vi "WLAN - niVST - OPPO - RFSG - Create and Down Load Wfm.vi"(0 "instrument handle":refnum<k15>="pxi1slot2", 1 "Waveform Generation Settings":T2 {"DSSS Data Rate (Mbps)" items=["1", "2", "5.5 CCK", "5.5 PBCC", "11 CCK", "11 PBCC", "22", "33"]; "OFDM Data Rate (Mbps)" items=["6", "9", "12", "18", "24", "36", "48", "54"]; "80211n PLCP Frame Format" items=["Mixed Format", "Greenfield Format"]; "Standard" items=["80211A/G/J/P OFDM", "80211B/G DSSS", "80211G DSSSOFDM", "80211N MIMOOFDM", "80211AC MIMOOFDM"]}, 5 "WaveformNamePostfix":string, 11 "error in":errorcluster, 12 "Address String":string="00:90:4C:C5:12:38") -> (4 "instrument handle":refnum<k15>, 6 "Rx_Test Parameters":T1 {"OFDM Data Rate (Mbps)" items=["6", "9", "12", "18", "24", "36", "48", "54"]; "DSSS Data Rate (Mbps)" items=["1", "2", "5.5 CCK", "5.5 PBCC", "11 CCK", "11 PBCC", "22", "33"]; "80211n PLCP Frame Format" items=["Mixed Format", "Greenfield Format"]}, 15 "error out":errorcluster)   [LabVIEW 2012]
uses:
  TV/RW/Includes/WLAN - TV - RW - INC - Rx_PER_Wfm_Settings.ctl
  TV/RW/Includes/WLAN - TV - RW - INC - RxTestParameters.ctl
  <instrlib>/niRFSG/niRFSG.llb/niRFSG Write Arb Waveform (Complex Input).vi
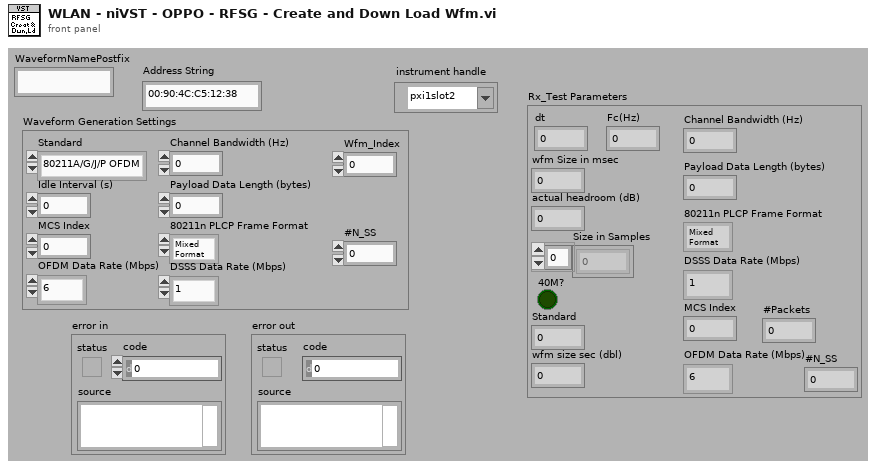
[diagram p1: front panel]
types:
  T1 = typedef "WLAN - TV - RW - INC - RxTestParameters.ctl" = cluster{"wfm Size in msec":i32, "actual headroom (dB)":dbl, "Size in Samples":i32[], "40M?":bool, "Standard ":i32, "wfm size sec (dbl)":dbl, "dt":dbl, "Channel Bandwidth (Hz)":dbl, "Payload Data Length (bytes)":i32, "80211n PLCP Frame Format":i32, "DSSS Data Rate (Mbps)":i32, "OFDM Data Rate (Mbps)":i32, "MCS Index":i32, "Fc(Hz)":dbl, "#Packets":i32, "#N_SS":i32}
  T2 = typedef "WLAN - TV - RW - INC - Rx_PER_Wfm_Settings.ctl" = cluster{"Standard":i32, "Channel Bandwidth (Hz)":dbl, "Idle Interval (s)":dbl, "MCS Index":i32, "80211n PLCP Frame Format":i32, "Payload Data Length (bytes)":i32, "OFDM Data Rate (Mbps)":i32, "DSSS Data Rate (Mbps)":i32, "Wfm_Index":i32, "#N_SS":i32}
  T3 = cluster{"Waveforms":cluster{"t0":dbl, "dt":dbl, "Y":cdb[]}[], "wfm Size in msec":i32, "actual headroom (dB)":dbl, "Size in Samples":i32[], "40M?":bool, "Standard ":i32, "wfm size sec (dbl)":dbl}
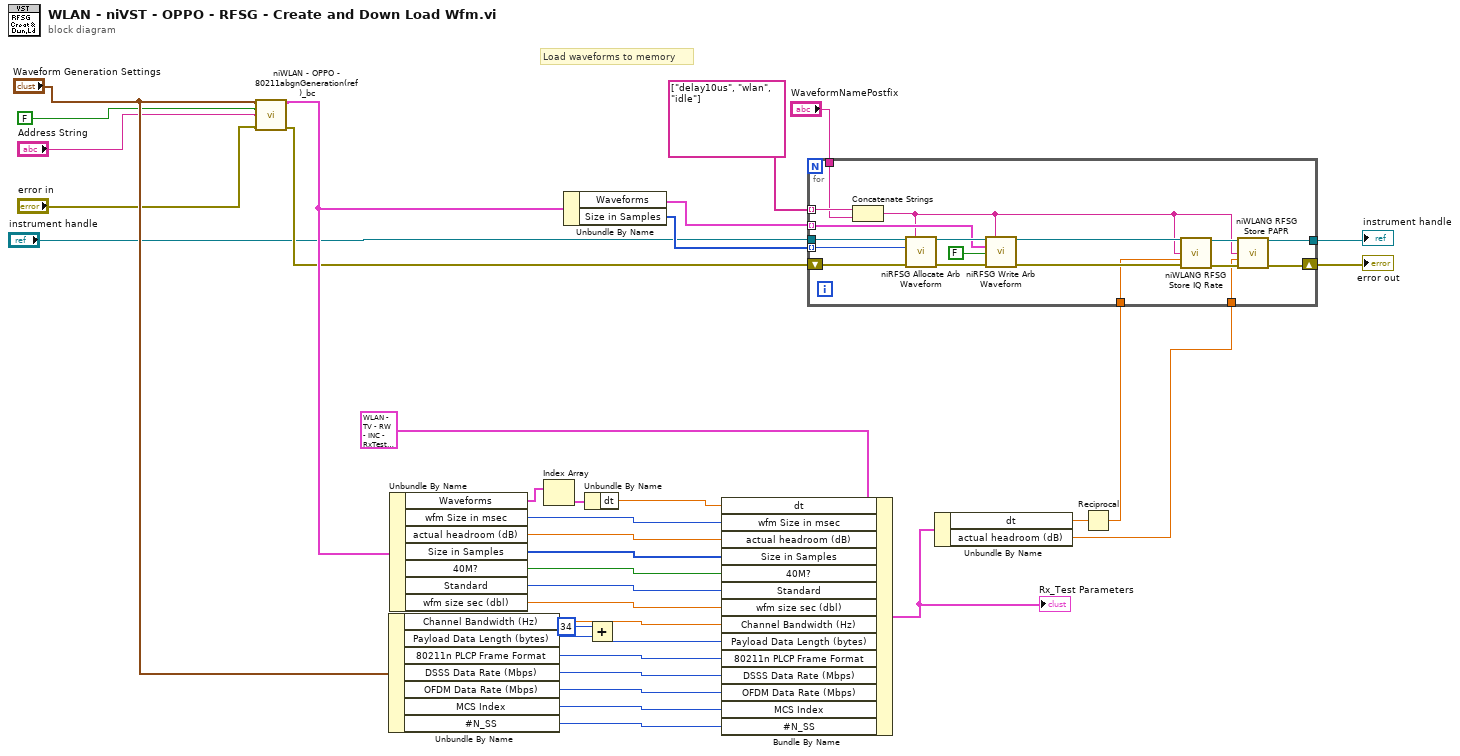
[diagram p0: block diagram]
diagram:
  # "Load waveforms to memory"
  n1 = call "niWLAN - OPPO - 80211abgnGeneration(ref)_bc.vi"("Rx Measurements Settings"="Waveform Generation Settings", "Without ACK ?"=FALSE ("w/ ACK"), "Address String"="Address String", "error in"="error in") -> ("Cluster"=w15:T3, "error out"=w14:errorcluster)  [unwired: 10 in]
  n2 = Unbundle By Name("Waveform Generation Settings") -> ("Channel Bandwidth (Hz)"=w26:dbl, "Payload Data Length (bytes)"=w25:i32, "80211n PLCP Frame Format"=w24:i32, "DSSS Data Rate (Mbps)"=w23:i32, "OFDM Data Rate (Mbps)"=w22:i32, "MCS Index"=w21:i32, "#N_SS"=w9:i32)
  n3 = Unbundle By Name(w15) -> ("Waveforms"=w35:cluster{"t0":dbl, "dt":dbl, "Y":cdb[]}[], "wfm Size in msec"=w32:i32, "actual headroom (dB)"=w28:dbl, "Size in Samples"=w29:i32[], "40M?"=w30:bool, "Standard"=w31:i32, "wfm size sec (dbl)"=w27:dbl)
  n4 = Index Array(array=w35) -> (element=w34:cluster{"t0":dbl, "dt":dbl, "Y":cdb[]})  [unwired: 1 in]
  n5 = Unbundle By Name(w15) -> ("Waveforms"=w16:cluster{"t0":dbl, "dt":dbl, "Y":cdb[]}[], "Size in Samples"=w17:i32[])
  n6 = Unbundle By Name(w34) -> ("dt"=w33:dbl)
  n7 = Add(x=34, y=w25) -> (x+y=w20:i32)
  n8 = Bundle By Name(cluster=T1 {"wfm Size in msec"=0, "actual headroom (dB)"=0.0, "Size in Samples"=[], "40M?"=FALSE, "Standard "=0, "wfm size sec (dbl)"=0.0, "dt"=0.0, "Channel Bandwidth (Hz)"=0.0, "Payload Data Length (bytes)"=0, "80211n PLCP Frame Format"=0, "DSSS Data Rate (Mbps)"=0, "OFDM Data Rate (Mbps)"=0, "MCS Index"=0, "Fc(Hz)"=0.0, "#Packets"=0, "#N_SS"=0} ("Cluster"), "dt"=w33, "wfm Size in msec"=w32, "actual headroom (dB)"=w28, "Size in Samples"=w29, "40M?"=w30, "Standard"=w31, "wfm size sec (dbl)"=w27, "Channel Bandwidth (Hz)"=w26, "Payload Data Length (bytes)"=w20, "80211n PLCP Frame Format"=w24, "DSSS Data Rate (Mbps)"=w23, "OFDM Data Rate (Mbps)"=w22, "MCS Index"=w21, "#N_SS"=w9) -> (w7:T1)
  "Rx_Test Parameters" <- w7
  n9 = Unbundle By Name(w7) -> ("dt"=w6:dbl, "actual headroom (dB)"=w2:dbl)
  n10 = Reciprocal(x=w6) -> (1/x=w3:dbl)
  n11 = for {
    tunnel: "instrument handle" -> [w50]
    shift-right: [w42] -> w5
    shift-left: w14 -> [w51]
    tunnel: string[] ["delay10us", "wlan", "idle"] -> [w48] mode=indexing
    tunnel: w17 -> [w49] mode=indexing
    tunnel: w16 -> [w46] mode=indexing
    tunnel: "WaveformNamePostfix" -> [w47]
    tunnel: [w40] -> w4
    tunnel: w3 -> [w38]
    tunnel: w2 -> [w37]
    n12 = Concatenate Strings(w48, w47) -> (w39:string)
    n13 = call <instrlib>:"niRFSG Allocate Arb Waveform.vi"("instrument handle"=w50, "name"=w39, "size in samples"=w49, "error in"=w51) -> ("instrument handle out"=w53:refnum<k15>, "error out"=w52:errorcluster)  [unwired: 10 in]
    n14 = call-poly <instrlib>:"niRFSG Write Arb Waveform.vi"("instrument handle"=w53, "name"=w39, "IQ waveform"=w46, "use waveform dt for IQ rate?"=FALSE, "error in"=w52) -> ("instrument handle out"=w41:refnum<k15>, "error out"=w43:errorcluster)  [unwired: 9 in]
    n15 = call <vilib>:"niWLANG RFSG Store IQ Rate.vi"("instrument handle"=w41, "waveform name"=w39, "IQ rate (S/s)"=w38, "error in"=w43) -> ("instrument handle out"=w44:refnum<k15>, "error out"=w45:errorcluster)  [unwired: 1 in, 9 out]
    n16 = call <vilib>:"niWLANG RFSG Store PAPR.vi"("instrument handle"=w44, "waveform name"=w39, "PAPR (dB)"=w37, "error in"=w45) -> ("instrument handle out"=w40:refnum<k15>, "error out"=w42:errorcluster)  [unwired: 10 out]
  }
  "error out" <- w5
  "instrument handle" <- w4
